vi "Read Coords.vi"(8 "error in (no error)":errorcluster, 11 "ShortcutMenuActivationMsg in":refnum<class "ShortcutMenuActivationMsg.lvclass">) -> (0 "error out":errorcluster, 2 "Coords":T1, 3 "ShortcutMenuActivationMsg out":refnum<class "ShortcutMenuActivationMsg.lvclass">)   [LabVIEW 2017, in "ActorEvents.lvlib" / "ShortcutMenuActivationMsg.lvclass"]
uses:
  ShortcutMenuActivationMsg.lvclass
  <vilib>/Utility/miscctls.llb/LVPoint32TypeDef.ctl
  ShortcutMenuActivationMsg.lvclass/ShortcutMenuActivationMsg.ctl
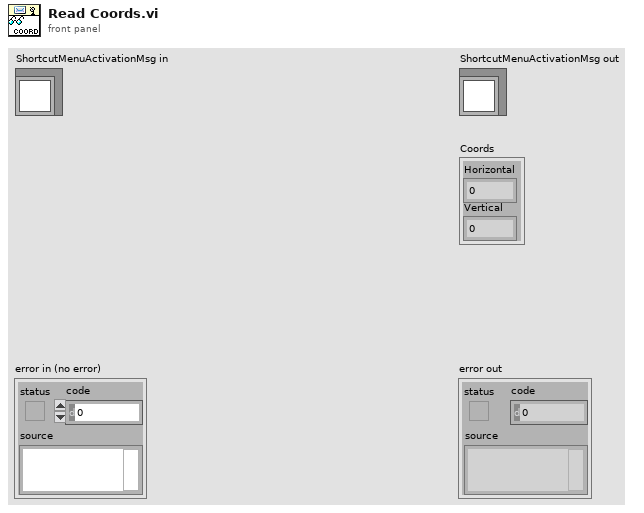
[diagram p1: front panel]
types:
  T1 = typedef "LVPoint32TypeDef.ctl" = cluster{"Horizontal":i32, "Vertical":i32}
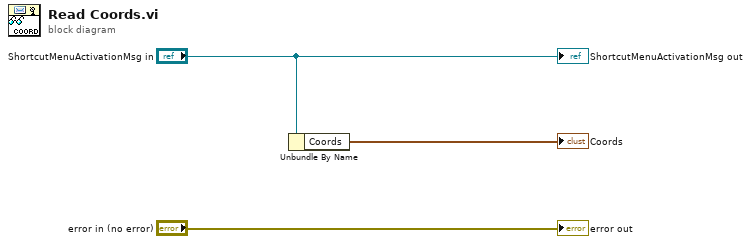
[diagram p0: block diagram]
diagram:
  n1 = Unbundle By Name("ShortcutMenuActivationMsg in") -> ("Coords"=→"Coords":T1)
  "error out" <- "error in (no error)"
  "ShortcutMenuActivationMsg out" <- "ShortcutMenuActivationMsg in"
